vi "clear buffer array.vi"(8 "error in (no error)":errorcluster, 10 "Image array":T1[](array[typedef]), 11 "ptr array":u64[](array[numeric])) -> (0 "error out":errorcluster)   [LabVIEW 2021, in "Camera.lvlib" / "Camera.lvclass"]
uses:
  Camera.lvclass
  <vilib>/vision/Image Controls.llb/IMAQ Image.ctl
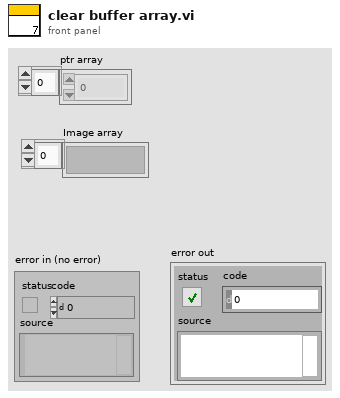
[diagram p1: front panel]
types:
  T1 = typedef "IMAQ Image.ctl" = refnum<image>
  T2 = enum32{"Map Pixel Pointer", "Unmap Pixel Pointer", "Get Pixels Infos"}
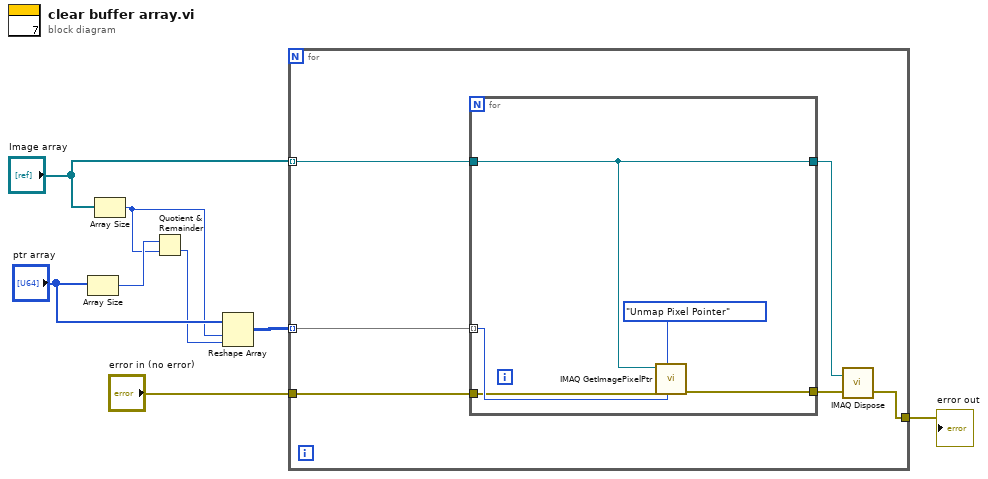
[diagram p0: block diagram]
diagram:
  n1 = Array Size(array="ptr array") -> (size(s)=w6:i32)
  n2 = Array Size(array="Image array") -> (size(s)=w3:i32)
  n3 = Quotient & Remainder(x=w6, y=w3) -> (floor(x/y)=w4:i32)  [unwired: 1 out]
  n4 = Reshape Array("ptr array", w3, w4) -> (w2:u64[][])
  n5 = for {
    tunnel: [w9] -> w8
    tunnel: "Image array" -> [w13] mode=indexing
    tunnel: w2 -> [w14] mode=indexing
    tunnel: "error in (no error)" -> [w12]
    n6 = for {
      tunnel: [w16] -> w10
      tunnel: w14 -> [w18] mode=indexing
      tunnel: w13 -> [w15]
      tunnel: w12 -> [w17]
      tunnel: [w15] -> w11
      n7 = call "IMAQ GetImagePixelPtr"("Pixel Pointer in"=w18, "Function"=T2."Unmap Pixel Pointer", "error in (no error)"=w17, "Image"=w15) -> ("error out"=w16:errorcluster)  [unwired: 2 in, 5 out]
    }
    n8 = call "IMAQ Dispose"("Image"=w11, "error in (no error)"=w10) -> ("error out"=w9:errorcluster)  [unwired: 4 in]
  }
  "error out" <- w8
